vi "VI Tree.vi"   [LabVIEW 2013, in "DmmPwr Simulator.lvlib"]
doc: "This is the instrument driver for the Dmm and power supply. The VI Tree displays all the user-callable VIs of the instrument driver in an organized table."
uses:
  <instrlib>/DmmPwr Simulator/DmmPwr Simulator.lvlib
panel:
  # "SEE DIAGRAM\nFOR VI TREE."
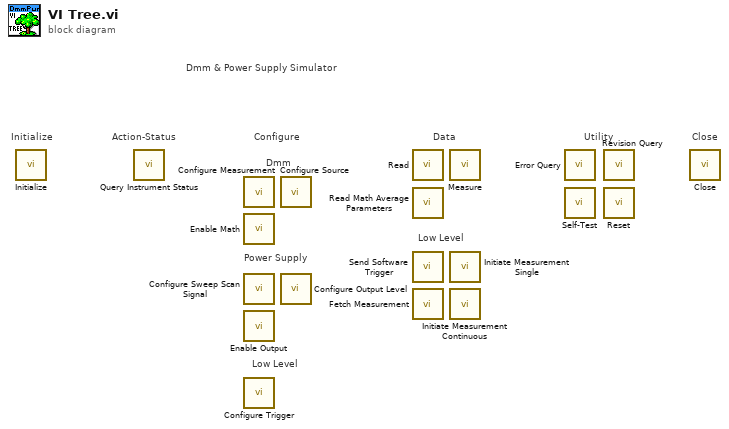
[diagram p0: block diagram]
diagram:
  # "Action-Status"
  # "Data"
  # "Power Supply"
  # "Dmm"
  # "Dmm & Power Supply Simulator"
  # "Low Level"
  # "Low Level"
  # "Configure"
  # "Utility"
  # "Close"
  # "Initialize"
  n1 = call <instrlib>:"Initialize.vi"() -> ()  [unwired: 10 in, 2 out]
  n2 = call <instrlib>:"Query Instrument Status.vi"() -> ()  [unwired: 9 in, 3 out]
  n3 = call <instrlib>:"Configure Measurement.vi"() -> ()  [unwired: 10 in, 2 out]
  n4 = call <instrlib>:"Enable Math.vi"() -> ()  [unwired: 10 in, 2 out]
  n5 = call <instrlib>:"Configure Sweep Scan Signal.vi"() -> ()  [unwired: 10 in, 2 out]
  n6 = call <instrlib>:"Enable Output.vi"() -> ()  [unwired: 10 in, 2 out]
  n7 = call <instrlib>:"Configure Trigger.vi"() -> ()  [unwired: 10 in, 2 out]
  n8 = call <instrlib>:"Configure Source.vi"() -> ()  [unwired: 10 in, 2 out]
  n9 = call <instrlib>:"Configure Output Level.vi"() -> ()  [unwired: 10 in, 2 out]
  n10 = call <instrlib>:"Read.vi"() -> ()  [unwired: 9 in, 3 out]
  n11 = call <instrlib>:"Read Math Average Parameters.vi"() -> ()  [unwired: 10 in, 6 out]
  n12 = call <instrlib>:"Send Software Trigger.vi"() -> ()  [unwired: 10 in, 2 out]
  n13 = call <instrlib>:"Fetch Measurement.vi"() -> ()  [unwired: 9 in, 3 out]
  n14 = call <instrlib>:"Measure.vi"() -> ()  [unwired: 9 in, 3 out]
  n15 = call <instrlib>:"Initiate Measurement Single.vi"() -> ()  [unwired: 10 in, 2 out]
  n16 = call <instrlib>:"Initiate Measurement Continuous.vi"() -> ()  [unwired: 10 in, 2 out]
  n17 = call <instrlib>:"Error Query.vi"() -> ()  [unwired: 8 in, 4 out]
  n18 = call <instrlib>:"Self-Test.vi"() -> ()  [unwired: 8 in, 4 out]
  n19 = call <instrlib>:"Revision Query.vi"() -> ()  [unwired: 8 in, 4 out]
  n20 = call <instrlib>:"Reset.vi"() -> ()  [unwired: 10 in, 2 out]
  n21 = call <instrlib>:"Close.vi"() -> ()  [unwired: 11 in, 1 out]
